vi "Thorlabs Z Translation Stage Module.vi"(7 "Action":T1, 8 "error in (no error)":errorcluster, 9 "Cluster In":T3, 10 "Set/Get":T2, 11 ".NET Refnum in":refnum<k24>) -> (0 "error out":errorcluster, 2 "Cluster out":T3, 3 ".NET Refnum out":refnum<k24>)   [LabVIEW 2018]
uses:
  C:/Project/SerialSectionOCT/SerialSectOCT/Labview Software/Thorlabs.MotionControl.Controls.dll
  Thorlabs.MotionControl.Controls.dll
  Hardware Mfg/Thorlabs Translation Stages/Controls/Translation Stage Cluster.ctl
  Controls/Translation Stage Types.ctl
  Controls/Set Get Controls.ctl
  Hardware Mfg/Thorlabs Translation Stages/Controls/Motion Translation Module Control2.ctl
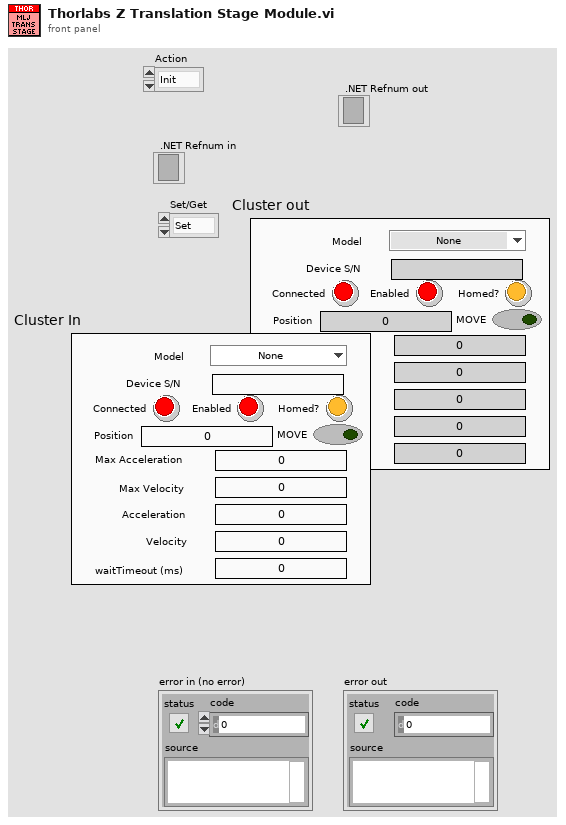
[diagram p1: front panel]
types:
  T1 = typedef "Motion Translation Module Control2.ctl" = enum16{"Init", "Home", "Status", "Velocity/Accel", "Position", "Jog", "Stop", "Uninit", "Enable", "Disable"}
  T2 = typedef "Set Get Controls.ctl" = enum16{"Set", "Get"}
  T3 = typedef "Translation Stage Cluster.ctl" = cluster{"Position":dbl, "Is.Enabled?":bool, "Is.Connected?":bool, "Device SN":string, "AccelerationMaximum":dbl, "VelocityMaximum":dbl, "Acceleration":dbl, "Velocity":dbl, "waitTimeout (ms)":i32, "Model":T4, "Is.Homed?":bool, "MOVE":bool}
  T4 = typedef "Translation Stage Types.ctl" = enum16{"None", "Thorlabs LTS", "Thorlabs MLJ"}
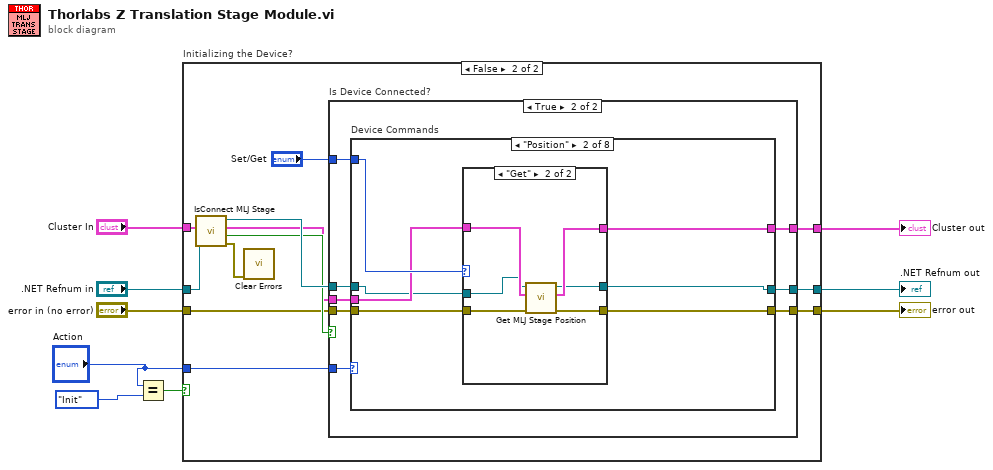
[diagram p0: block diagram]
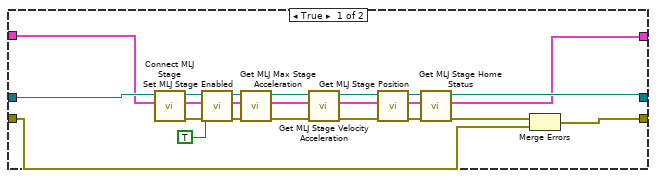
[diagram p2: hidden frame]
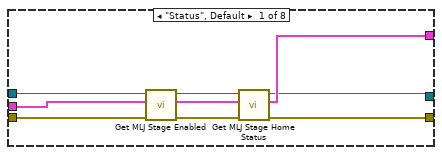
[diagram p4: hidden frame]
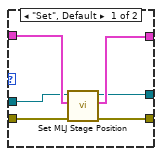
[diagram p5: hidden frame]
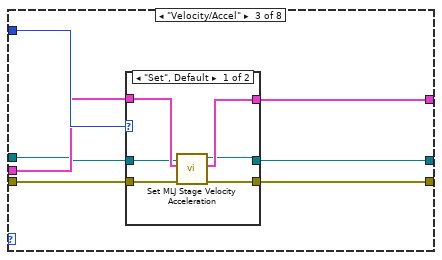
[diagram p6: hidden frame]
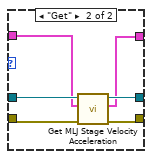
[diagram p7: hidden frame]
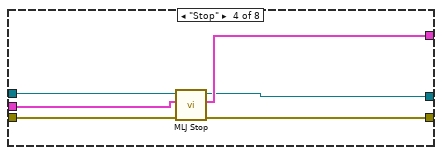
[diagram p8: hidden frame]
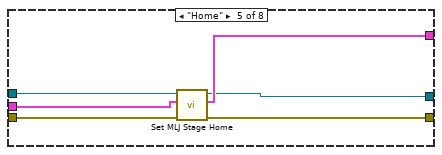
[diagram p9: hidden frame]
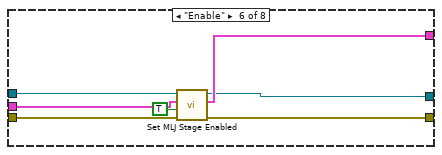
[diagram p10: hidden frame]
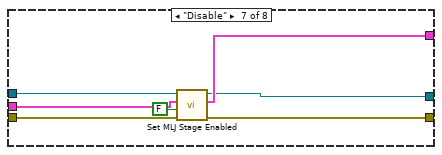
[diagram p11: hidden frame]
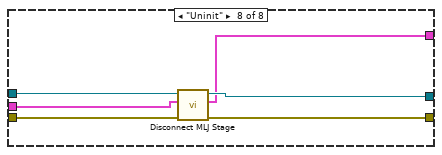
[diagram p12: hidden frame]
diagram:
  n1 = Equal?(x="Action", y=Motion_Translation_Module_Control2."Init" ("Action")) -> (x = y?=w3:bool)
  n2 = case "Initializing the Device?" shown="False" w3 {
    tunnel: ".NET Refnum in" -> [w32 w39]
    tunnel: [w19 w44] -> w8
    tunnel: [w18 w43] -> w7
    tunnel: [w16 w42] -> w6
    tunnel: "error in (no error)" -> [w15 w33]
    tunnel: "Cluster In" -> [w31 w37]
    tunnel: "Action" -> [_ w41]
    frame True {
      n3 = call "Connect MLJ Stage.vi"("Cluster in"=w31, "MLJ Reference In"=w32) -> ("error out"=w30:errorcluster, "Cluster out"=w28:T3, "MLJ Reference Out"=w29:refnum<k24>)  [unwired: 6 in, 1 out]
      n4 = call "Set MLJ Stage Enabled.vi"("error in (no error)"=w30, "Enable/Disable"=TRUE, "Cluster in"=w28, "MLJ Reference In"=w29) -> ("error out"=w27:errorcluster, "Cluster out"=w26:T3, "MLJ Reference Out"=w25:refnum<k24>)  [unwired: 5 in]
      n5 = call "Get MLJ Max Stage Acceleration.vi"("error in (no error)"=w27, "Cluster in"=w26, "MLJ Reference In"=w25) -> ("error out"=w24:errorcluster, "Cluster out"=w13:T3, "MLJ Reference Out"=w11:refnum<k24>)  [unwired: 6 in]
      n6 = call "Get MLJ Stage Velocity Acceleration.vi"("error in (no error)"=w24, "Cluster in"=w13, ".NET Refnum in"=w11) -> ("error out"=w14:errorcluster, "Cluster out"=w12:T3, ".NET Refnum in"=w10:refnum<k24>)  [unwired: 5 in, 1 out]
      n7 = call "Get MLJ Stage Position.vi"("error in (no error)"=w14, "Cluster in"=w12, "MLJ Reference In"=w10) -> ("error out"=w23:errorcluster, "Cluster out"=w21:T3, "MLJ Reference Out"=w20:refnum<k24>)  [unwired: 5 in, 1 out]
      n8 = call "Get MLJ Stage Home Status.vi"("error in (no error)"=w23, "Cluster in"=w21, "MLJ Reference In"=w20) -> ("error out"=w22:errorcluster, "Cluster out"=w18:T3, "MLJ Reference Out"=w19:refnum<k24>)  [unwired: 6 in]
      n9 = Merge Errors(w22, w15) -> (w16:errorcluster)
    }
    frame False {
      n10 = call "IsConnect MLJ Stage.vi"("Cluster in"=w37, "MLJ Reference In"=w39) -> ("error out"=w34:errorcluster, "IsConnected"=w36:bool, "Cluster out"=w35:T3, "MLJ Reference Out"=w38:refnum<k24>)  [unwired: 6 in]
      n11 = call <vilib>:"Clear Errors.vi"("error in (no error)"=w34) -> ()  [unwired: 5 in, 2 out]
      n12 = case "Is Device Connected?" shown="True" w36 {
        tunnel: w38 -> [w45 w55]
        tunnel: [w45 w54] -> w44
        tunnel: [w47 w53] -> w43
        tunnel: [w46 w52] -> w42
        tunnel: w33 -> [w46 w51]
        tunnel: "Set/Get" -> [_ w50]
        tunnel: w41 -> [_ w49]
        tunnel: w35 -> [w47 w48]
        frame False {
        }
        frame True {
          n13 = case "Device Commands" shown="\"Position\"" w49 {
            tunnel: w50 -> [_ w71 w90 _ _ _ _ _]
            tunnel: w48 -> [w57 w68 w87 w106 w112 w119 w126 w131]
            tunnel: w51 -> [w58 w70 w89 w108 w114 w121 w128 w134]
            tunnel: [w59 w66 w85 w104 w110 w117 w124 w132] -> w54
            tunnel: [w64 w69 w88 w107 w113 w120 w127 w133] -> w52
            tunnel: [w60 w67 w86 w105 w111 w118 w125 w130] -> w53
            tunnel: w55 -> [w56 w65 w84 w103 w109 w116 w123 w129]
            frame "Status", Default {
              n14 = call "Get MLJ Stage Enabled.vi"("error in (no error)"=w58, "Cluster in"=w57, "MLJ Reference In"=w56) -> ("error out"=w63:errorcluster, "Cluster out"=w62:T3, "MLJ Reference Out"=w61:refnum<k24>)  [unwired: 5 in, 1 out]
              n15 = call "Get MLJ Stage Home Status.vi"("error in (no error)"=w63, "Cluster in"=w62, "MLJ Reference In"=w61) -> ("error out"=w64:errorcluster, "Cluster out"=w60:T3, "MLJ Reference Out"=w59:refnum<k24>)  [unwired: 6 in]
            }
            frame "Position" {
              n16 = case shown="\"Get\"" w71 {
                tunnel: w70 -> [w77 w83]
                tunnel: [w76 w82] -> w69
                tunnel: w68 -> [w75 w81]
                tunnel: [w74 w80] -> w67
                tunnel: w65 -> [w73 w79]
                tunnel: [w72 w78] -> w66
                frame "Set", Default {
                  n17 = call "Set MLJ Stage Position.vi"("error in (no error)"=w77, "Cluster in"=w75, "LTS Reference In"=w73) -> ("error out"=w76:errorcluster, "Cluster out"=w74:T3, "LTS Reference Out"=w72:refnum<k24>)  [unwired: 6 in]
                }
                frame "Get" {
                  n18 = call "Get MLJ Stage Position.vi"("error in (no error)"=w83, "Cluster in"=w81, "MLJ Reference In"=w79) -> ("error out"=w82:errorcluster, "Cluster out"=w80:T3, "MLJ Reference Out"=w78:refnum<k24>)  [unwired: 5 in, 1 out]
                }
              }
            }
            frame "Velocity/Accel" {
              n19 = case shown="\"Set\", Default" w90 {
                tunnel: w89 -> [w96 w102]
                tunnel: [w95 w101] -> w88
                tunnel: w87 -> [w93 w98]
                tunnel: [w94 w97] -> w86
                tunnel: w84 -> [w92 w99]
                tunnel: [w91 w100] -> w85
                frame "Set", Default {
                  n20 = call "Set MLJ Stage Velocity Acceleration.vi"("error in (no error)"=w96, "Cluster in"=w93, "MLJ Reference In"=w92) -> ("error out"=w95:errorcluster, "Cluster out"=w94:T3, "MLJ Reference Out"=w91:refnum<k24>)  [unwired: 6 in]
                }
                frame "Get" {
                  n21 = call "Get MLJ Stage Velocity Acceleration.vi"("error in (no error)"=w102, "Cluster in"=w98, ".NET Refnum in"=w99) -> ("error out"=w101:errorcluster, "Cluster out"=w97:T3, ".NET Refnum in"=w100:refnum<k24>)  [unwired: 5 in, 1 out]
                }
              }
            }
            frame "Stop" {
              n22 = call "MLJ Stop.vi"("error in (no error)"=w108, "Cluster in"=w106, "MLJ Reference In"=w103) -> ("error out"=w107:errorcluster, "Cluster out"=w105:T3, "MLJ Reference Out"=w104:refnum<k24>)  [unwired: 6 in]
            }
            frame "Home" {
              n23 = call "Set MLJ Stage Home.vi"("error in (no error)"=w114, "Cluster in"=w112, "MLJ Reference In"=w109) -> ("error out"=w113:errorcluster, "Cluster out"=w111:T3, "MLJ Reference Out"=w110:refnum<k24>)  [unwired: 6 in]
            }
            frame "Enable" {
              n24 = call "Set MLJ Stage Enabled.vi"("error in (no error)"=w121, "Enable/Disable"=TRUE, "Cluster in"=w119, "MLJ Reference In"=w116) -> ("error out"=w120:errorcluster, "Cluster out"=w118:T3, "MLJ Reference Out"=w117:refnum<k24>)  [unwired: 5 in]
            }
            frame "Disable" {
              n25 = call "Set MLJ Stage Enabled.vi"("error in (no error)"=w128, "Enable/Disable"=FALSE, "Cluster in"=w126, "MLJ Reference In"=w123) -> ("error out"=w127:errorcluster, "Cluster out"=w125:T3, "MLJ Reference Out"=w124:refnum<k24>)  [unwired: 5 in]
            }
            frame "Uninit" {
              n26 = call "Disconnect MLJ Stage.vi"("error in (no error)"=w134, "Cluster in"=w131, "MLJ Reference In"=w129) -> ("error out"=w133:errorcluster, "Cluster out"=w130:T3, "MLJ Reference Out"=w132:refnum<k24>)  [unwired: 6 in]
            }
          }
        }
      }
    }
  }
  ".NET Refnum out" <- w8
  "Cluster out" <- w7
  "error out" <- w6
